vi "WPI_ERRNoFreeCounter.vi"(11 "error in (no error)":errorcluster) -> (3 "CounterAllocation":errorcluster)   [LabVIEW 2017]
doc: "This software is licensed. Open the labview\\readme\\WPI Robotics Library Open Source License.txt file for more information."
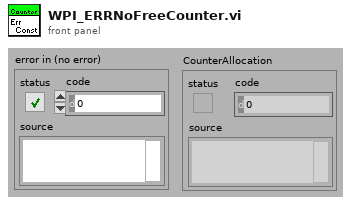
[diagram p1: front panel]
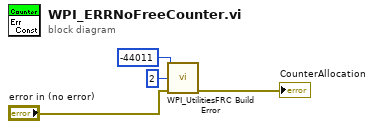
[diagram p0: block diagram]
diagram:
  n1 = call <vilib>:"WPI_UtilitiesFRC Build Error.vi"("error code"=-44011 ("code"), "chain levels to remove (1)"=2, "error in (no error)"="error in (no error)") -> ("error out"=→"CounterAllocation":errorcluster)  [unwired: 2 in, 10 out]
